vi "Field Draw Paths.vi"(4 "Draw Targets?":T2, 6 "Lado":enum16{"Esquerdo", "Direito"}(ring), 8 "Offset":T1, 9 "Scale mm/pixel":dbl, 10 "our_robots":T3[](array[typedef]), 11 "picture in":picture) -> (3 "picture out":picture)   [LabVIEW 2018]
uses:
  Core/AI Robot.ctl
  Intel/Functions Enum.ctl
  Intel/AttackerStates.ctl
  Path Planning/RRT/PathDests.ctl
  Path Planning/RRT/PathDest.ctl
  DrawTargets.ctl
  <vilib>/Utility/miscctls.llb/LVBoundsTypeDef.ctl
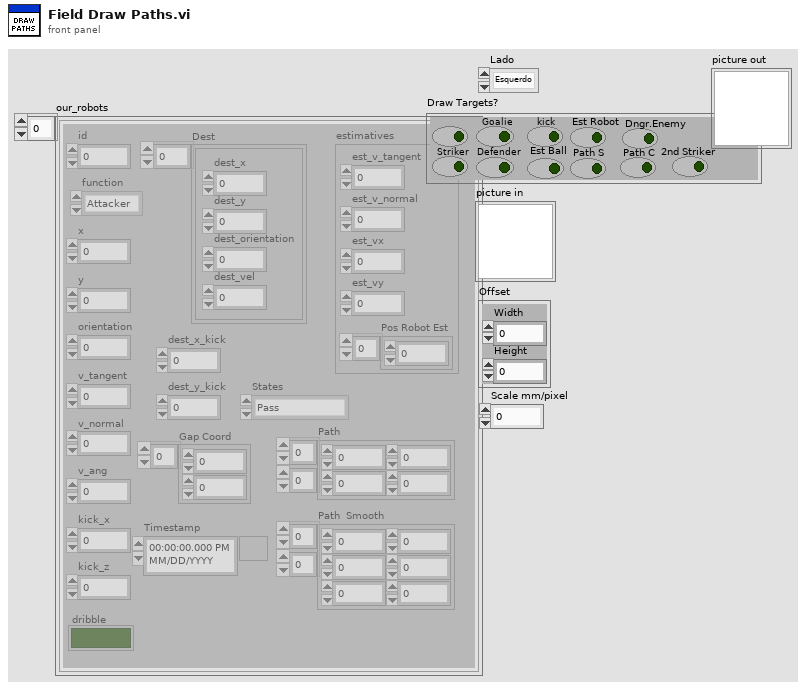
[diagram p1: front panel]
types:
  T1 = typedef "LVBoundsTypeDef.ctl" = cluster{"Width":u32, "Height":u32}
  T2 = typedef "DrawTargets.ctl" = cluster{"Attacker":bool, "Striker":bool, "Goalie":bool, "Defender":bool, "kick":bool, "Est Ball":bool, "Est Robot":bool, "Path S":bool, "Path C":bool, "Dngr.Enemy":bool, "2nd Striker":bool}
  T3 = typedef "AI Robot.ctl" = cluster{"id":u32, "function":T4, "x":dbl, "y":dbl, "orientation":dbl, "v_tangent":dbl, "v_normal":dbl, "v_ang":dbl, "kick_x":dbl, "kick_z":dbl, "dribble":bool, "Timestamp":timestamp, "estimatives":cluster{"est_v_tangent":dbl, "est_v_normal":dbl, "est_vx":dbl, "est_vy":dbl, "Pos Robot Est":dbl[]}, "dest_x_kick":dbl, "dest_y_kick":dbl, "Gap Coord":dbl[], "States":T5, "Path ":dbl[][], "Path  Smooth":dbl[][], "Dest":T6}
  T4 = typedef "Functions Enum.ctl" = enum16{"2nd Striker", "Attacker", "Goalie", "Defender", "Striker", "Goto 0", "Dummy", "Kicker", "ZigZag 0", "ZigZag 1", "ZigZag 2", "ZigZag 3", "ZigZag 4", "ZigZag 5", "ZigZag 6", "ZigZag 7", "ZigZag 8", ""}
  T5 = typedef "AttackerStates.ctl" = enum16{"Pass", "GoToTangent", "BallGetting", "GoToKick", ""}
  T6 = typedef "PathDests.ctl" = T7[]
  T7 = typedef "PathDest.ctl" = cluster{"dest_x":dbl, "dest_y":dbl, "dest_orientation":dbl, "dest_vel":dbl}
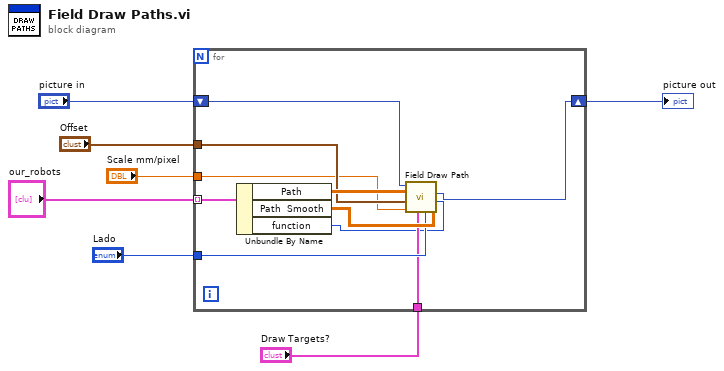
[diagram p0: block diagram]
diagram:
  n1 = for {
    tunnel: "our_robots" -> [w17] mode=indexing
    tunnel: "Lado" -> [w14]
    tunnel: "Draw Targets?" -> [w13]
    tunnel: "Offset" -> [w11]
    tunnel: "Scale mm/pixel" -> [w10]
    shift-right: [w9] -> w1
    shift-left: "picture in" -> [w12]
    n2 = Unbundle By Name(w17) -> ("Path"=w16:dbl[][], "Path  Smooth"=w15:dbl[][], "function"=w8:T4)
    n3 = call "Field Draw Path.vi"("Pontos Smooth"=w15, "function"=w8, "Lado"=w14, "Draw Targets?"=w13, "Scale mm/pixel"=w10, "Offset"=w11, "Pontos"=w16, "picture in"=w12) -> ("picture out"=w9:picture)  [unwired: 3 in]
  }
  "picture out" <- w1
